vi "ArrayToTable2(SubVI).vi"(11 "Table1D":sgl[](array[numeric])) -> (1 "Size":i32, 3 "String":string)   [LabVIEW 2017, in "LV_Unicorn.lvlib"]
uses:
  LV_Unicorn.lvlib
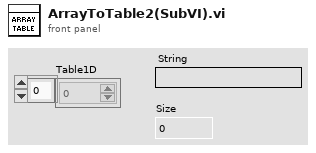
[diagram p1: front panel]
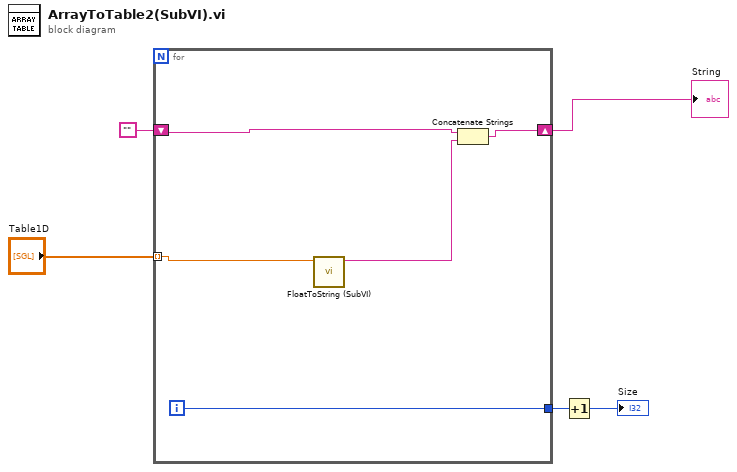
[diagram p0: block diagram]
diagram:
  n1 = for {
    tunnel: "Table1D" -> [w10] mode=indexing
    shift-right: [w7] -> w5
    shift-left: "" -> [w9]
    tunnel: [w6] -> w2
    i -> [w6]
    n2 = call "FloatToString (SubVI).vi"("Numeric"=w10) -> ("String"=w8:string)  [unwired: 10 in]
    n3 = Concatenate Strings(w9, w8) -> (w7:string)
  }
  "String" <- w5
  n4 = Increment(x=w2) -> (x+1=→"Size":i32)
